vi "subRotateQuat.vi"(10 "dotToTotate":dbl[](array[numeric]), 11 "q":dbl[](array[numeric])) -> (3 "qRotated":dbl[](array[numeric]))   [LabVIEW 2020]
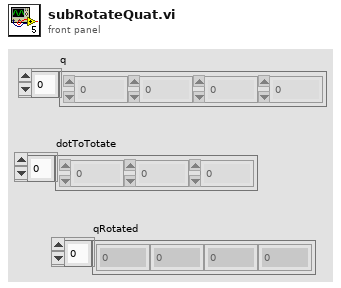
[diagram p1: front panel]
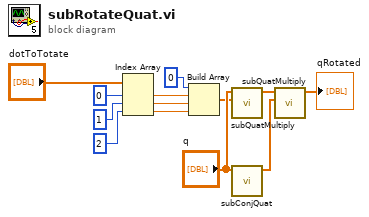
[diagram p0: block diagram]
diagram:
  n1 = Index Array(array="dotToTotate", index #1=0, index #2=1, index #3=2) -> (element #1=w7:dbl, element #2=w6:dbl, element #3=w5:dbl)
  n2 = Build Array(0, w7, w6, w5) -> (w1:dbl[])
  n3 = call "subQuatMultiply.vi"("q2"=w1, "q1"="q") -> ("qResult"=w12:dbl[])  [unwired: 9 in]
  n4 = call "subConjQuat.vi"("q"="q") -> ("qConj"=w11:dbl[])  [unwired: 10 in]
  n5 = call "subQuatMultiply.vi"("q2"=w11, "q1"=w12) -> ("qResult"=→"qRotated":dbl[])  [unwired: 9 in]
